vi "Write Do.vi"(0 "FPGA API in":refnum<class "FPGA API Mock.lvclass">, 5 "#DO":T1 items=["DO 0 [KP1] [M12]", "DO 1 [ON KP2] [M21]", "DO 2 [ON KP3] [M24]", "DO 3 [WATER Y18.1 [DO3]]", "DO 4 [WATER Y18.2 [DO4]]", "DO 5 [KP6 Y29.1 33.7]", "DO 6 [KP7 Y29.2 33.8]", "DO 7 [KP8 Y29.3 33.9]", "DO 8 [KP9 Y29.4  33.12]", "DO 9 [KP10 Y29.5 33.1]", "DO 10 [KP11 Y29.6 33.2]", "DO 11 [KP12 Y29.7  33.13]", "DO 12 [KP13 Y29.8  33.11]", "DO 13 [KP14 Y29.9 33.10]", "DO 14 [KP15 Y29.10  33.6]", "DO 15 [KP16 Y29.11  33.5]", "DO 16 [KP17 Y29.12  33.4]", "DO 17 [KP18 Y29.13 33.3]", "DO 18 [AIR KP19]", "DO 19 [STEP DRIVE EN KP20]", "DO 20 [KP21 Y44.1 OPEN]", "DO 21 [ KP22 Y44.1 CLOSE]", "DO 22 [ KP23 Y44.2 OPEN]", "DO 23", "DO 24 [STEP DRIVE 1]", "DO 25 [STEP DRIVE 2]"], 7 "value":bool, 9 "Time uSec":u32, 11 "error in (no error)":errorcluster) -> (4 "FPGA API out":refnum<class "FPGA API Mock.lvclass">, 15 "error out":errorcluster)   [LabVIEW 2019, in "FPGA API Mock.lvclass"]
uses:
  FPGA API Mock.lvclass
  FPGA/TypeDef/DO index.ctl
  FPGA API Mock.lvclass/FPGA API Mock.ctl
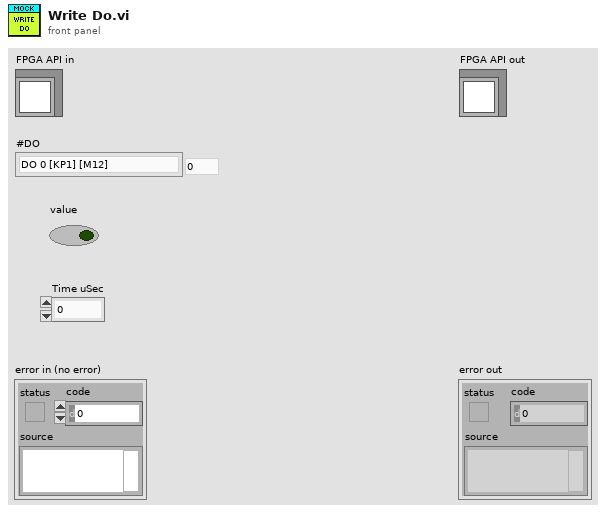
[diagram p1: front panel]
types:
  T1 = typedef "DO index.ctl" = u8
  T2 = typedef "FPGA API Mock.lvclass/Data.ctl" = cluster{"DO":bool[], "DI":bool[], "AI":dbl[], "AO":dbl[]}
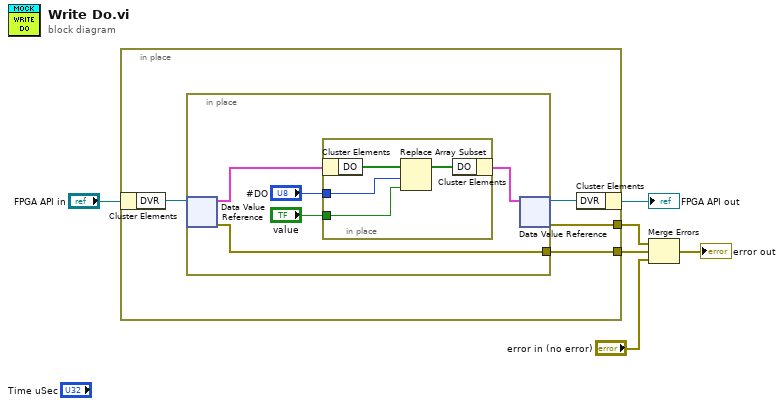
[diagram p0: block diagram]
diagram:
  n1 = in-place {
    in-place-border: [w8] -> w2
    in-place-border: [w7] -> w1
    n2 = in-place-cluster #1("FPGA API in") -> ("DVR"=w10:refnum<data-value>)
    n3 = in-place {
      in-place-border: [w11] -> w7
      n4 = in-place-dvr #2(w10) -> (w13:T2, w11:errorcluster)
      n5 = in-place {
        in-place-border: "#DO" -> [w17]
        in-place-border: "value" -> [w16]
        n6 = in-place-cluster #3(w13) -> ("DO"=w19:bool[])
        n7 = Replace Array Subset(array=w19, new element=w16, index=w17) -> (w18:bool[])
        n8 = in-place-cluster #3("DO"=w18) -> (w12:T2)
      }
      n9 = in-place-dvr #2(w12) -> (w9:refnum<data-value>, w8:errorcluster)
    }
    n10 = in-place-cluster #1("DVR"=w9) -> (→"FPGA API out":refnum<class "FPGA API Mock.lvclass">)
  }
  n11 = Merge Errors(w2, w1, "error in (no error)") -> (→"error out":errorcluster)
